vi "Case_structure_with_switch.vi"() -> ()   [LabVIEW 2020]
panel:
  in  "Numeric":dbl
  in  "stop":bool
  out "Thermometer":dbl(slide) scale=0.0..100.0
  in  "Temperature":dbl(slide) scale=0.0..100.0
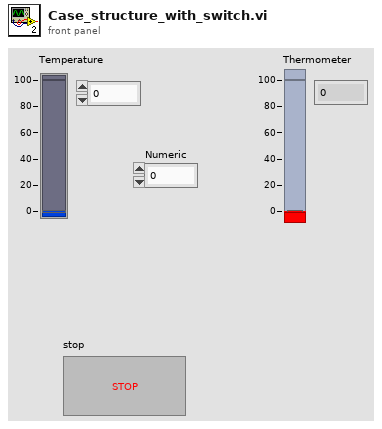
[diagram p1: front panel]
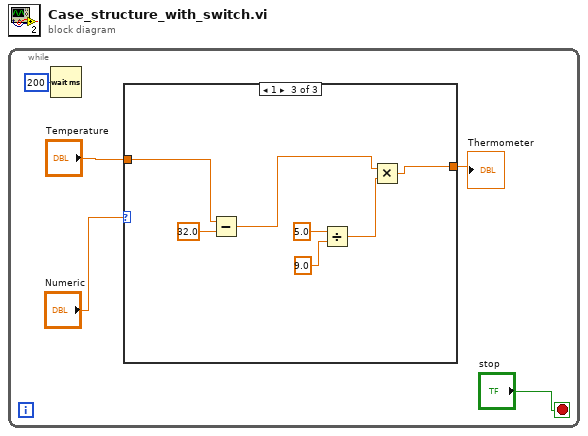
[diagram p0: block diagram]
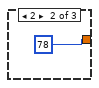
[diagram p3: hidden frame]
diagram:
  n1 = while {
    stop <- "stop" stop-if-true
    n2 = Wait (ms)(milliseconds to wait=200) -> ()  [unwired: 1 out]
    n3 = case shown="1" "Numeric" {
      tunnel: "Temperature" -> [w6 _ w9]
      tunnel: [w6 78 w8] -> w4
      frame 0, Default {
      }
      frame 2 {
      }
      frame 1 {
        n4 = Subtract(x=w9, y=32.0) -> (x-y=w10:dbl)
        n5 = Divide(x=5.0, y=9.0) -> (x/y=w11:dbl)
        n6 = Multiply(x=w10, y=w11) -> (x*y=w8:dbl)
      }
    }
    "Thermometer" <- w4
  }
